vi "Emit Beep.vi"(8 "error in (no error)":errorcluster, 9 "Beep Duration (.25 s)":dbl=0.25, 10 "Beep Frequency (300)":dbl=300.0, 11 "VISA resource name":refnum<visa-resource-name>) -> (0 "error out":errorcluster, 3 "VISA resource name out":refnum<visa-resource-name>)   [LabVIEW 2021, in "Keithley 2450.lvlib"]
doc: "Emits a beep of a user defined frequency and duration."
uses:
  Keithley 2450.lvlib
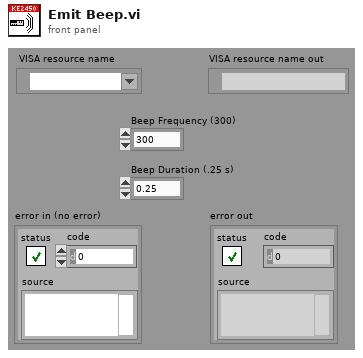
[diagram p1: front panel]
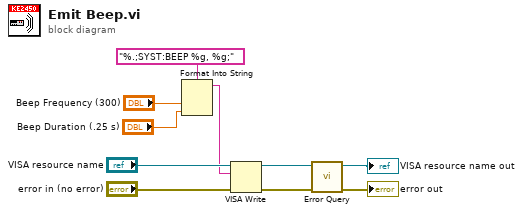
[diagram p0: block diagram]
diagram:
  n1 = Format Into String(format string="%.;SYST:BEEP %g, %g;", "Beep Frequency (300)", "Beep Duration (.25 s)") -> (resulting string=w4:string)  [unwired: 2 in, 1 out]
  n2 = VISA Write(VISA resource name="VISA resource name", write buffer=w4, error in (no error)="error in (no error)") -> (VISA resource name out=w8:refnum<visa-resource-name>, error out=w5:errorcluster)  [unwired: 1 out]
  n3 = call "Error Query.vi"("error in (no error)"=w5, "VISA resource name"=w8) -> ("error out"=→"error out":errorcluster, "VISA resource name out"=→"VISA resource name out":refnum<visa-resource-name>)  [unwired: 8 out]
